vi "backwards difference.vi"   [LabVIEW 2009, in "common.lvlib"]
uses:
  common.lvlib
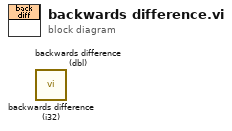
[diagram p0: block diagram]
diagram:
  n1 = call "backwards difference (i32).vi"() -> ()  [unwired: 3 in, 1 out]
  n2 = call "backwards difference (dbl).vi"() -> ()  [unwired: 3 in, 1 out]
